vi "Get Owning Project Path.vi"(8 "error in (no error)":errorcluster) -> (0 "error out":errorcluster, 2 "Path":path)   [LabVIEW 2019, in "Project Sync Tools.lvclass"]
uses:
  Project Sync Tools.lvclass
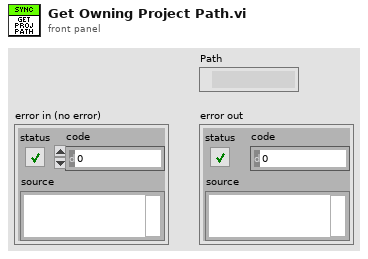
[diagram p1: front panel]
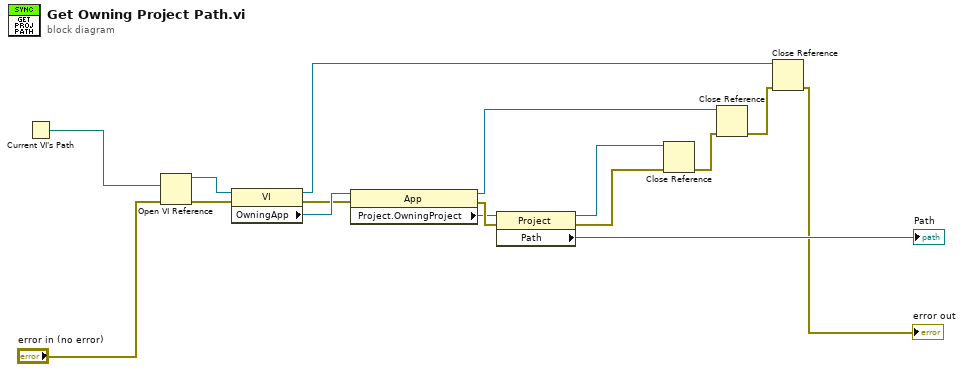
[diagram p0: block diagram]
diagram:
  n1 = Current VI's Path() -> (path=w12:path)
  n2 = Open VI Reference(vi path=w12, error in (no error)="error in (no error)") -> (vi reference=w11:refnum<vi>, error out=w10:errorcluster)  [unwired: 4 in]
  n3 = property class="VI"(reference=w11, error in=w10) -> (reference out=w7:refnum<vi>, error out=w8:errorcluster, "OwningApp"=w9:refnum<vi>)
  n4 = property class="App"(reference=w9, error in=w8) -> (reference out=w6:refnum<vi>, error out=w14:errorcluster, "Project.OwningProject"=w13:refnum<vi>)
  n5 = property class="Project"(reference=w13, error in=w14) -> (reference out=w5:refnum<vi>, error out=w4:errorcluster, "Path"=→"Path":path)
  n6 = Close Reference(reference=w5, error in (no error)=w4) -> (error out=w3:errorcluster)
  n7 = Close Reference(reference=w6, error in (no error)=w3) -> (error out=w2:errorcluster)
  n8 = Close Reference(reference=w7, error in (no error)=w2) -> (error out=→"error out":errorcluster)
